vi "KlingerV2 Enable.vi"(4 "UnitDem":u8(ring) items=["Pas", "mm", "ps", "Degré (°)"], 5 "error in":errorcluster, 6 "Axe":u8(ring) items=["W", "X", "Y", "Z"], 7 "Enable":bool, 8 "VISA Rsrc":refnum<visa-resource-name>="SR530") -> (0 "error out":errorcluster, 1 "Position":dbl format="%#.1f", 2 "Ind Comm":string, 3 "Statut":bool)   [LabVIEW 2012]
doc: "Ce Vi définit la position actuelle de l'axe spécifié comme zéro."
panel:
  out "Message D'erreur":string
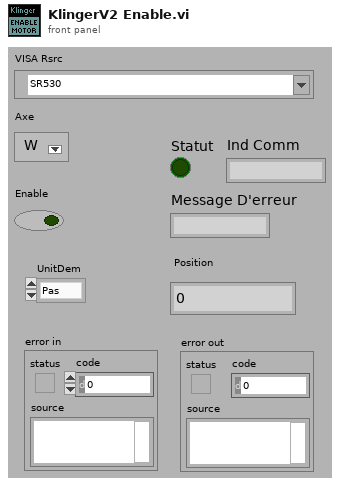
[diagram p1: front panel]
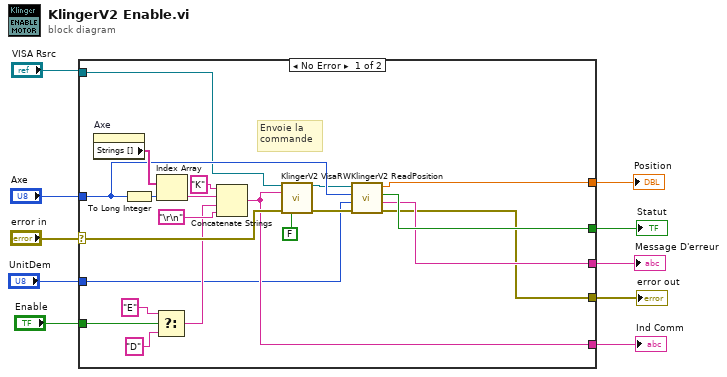
[diagram p0: block diagram]
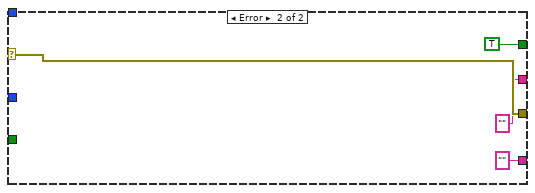
[diagram p2: hidden frame]
diagram:
  n1 = case shown="No Error" "error in" {
    selector: "error in" -> [w21 w35]
    tunnel: [w20 ""] -> w10
    tunnel: "Axe" -> [w25 _]
    tunnel: [w27 TRUE ("Statut")] -> w8
    tunnel: [w18 w35] -> w7
    tunnel: [w26 "" ("Message D'erreur")] -> w6
    tunnel: "VISA Rsrc" -> [w22 _]
    tunnel: "Enable" -> [w17 _]
    tunnel: [w12 _] -> w2
    tunnel: "UnitDem" -> [w11 _]
    frame No Error {
      # "Envoie la \ncommande"
      n2 = property on="Axe" class="Ring (strict)"() -> ("Strings []"=w30:string[])  [unwired: 2 in, 2 out]
      n3 = To Long Integer(number=w25) -> (32bit integer=w29:i32)
      n4 = Select(t="E", s=w17, f="D") -> (s? t:f=w13:string)
      n5 = Index Array(array=w30, index=w29) -> (element=w28:string)
      n6 = Concatenate Strings("K", w28, w13, "\r\n") -> (w20:string)
      n7 = call <userlib>:"KlingerV2 VisaRW.vi"("VISA Rsrc"=w22, "ChaineCom"=w20, "error in (no error)"=w21, "Lecture?(T)"=FALSE) -> ("VISA Rsrc Out"=w24:refnum<visa-resource-name>, "error out"=w23:errorcluster)  [unwired: 7 in, 3 out]
      n8 = call <userlib>:"KlingerV2 ReadPosition.vi"("error in"=w23, "UnitDem"=w11, "Axe"=w25, "VISA Rsrc"=w24) -> ("error out"=w18:errorcluster, "Cont Error"=w26:string, "Statut"=w27:bool, "Position"=w12:dbl)  [unwired: 1 in, 3 out]
    }
    frame Error {
    }
  }
  "error out" <- w7
  "Ind Comm" <- w10
  "Message D'erreur" <- w6
  "Statut" <- w8
  "Position" <- w2
